vi "SCP_command_filtering.vi"(11 "Input":string) -> (3 "concatenated string":string)   [LabVIEW 2018, in "SCP.lvlib"]
uses:
  SCP.lvlib
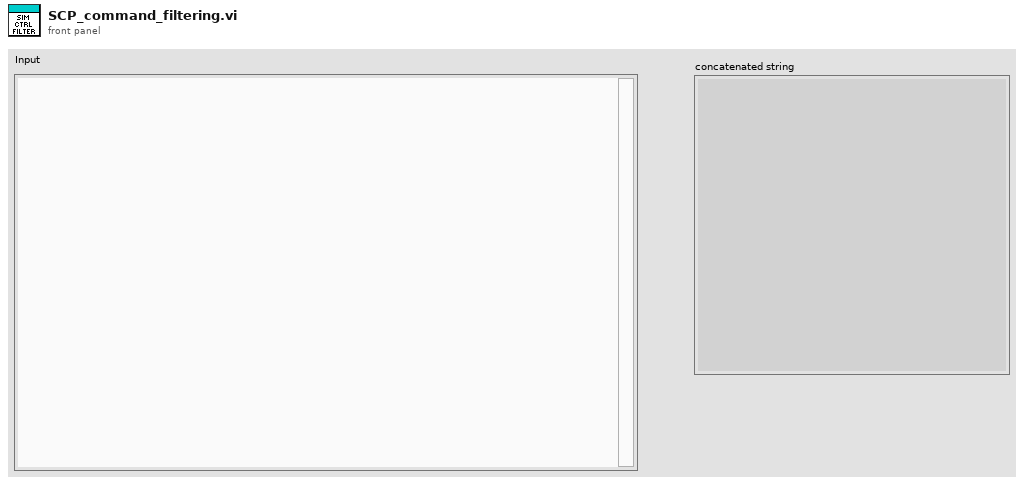
[diagram p1: front panel]
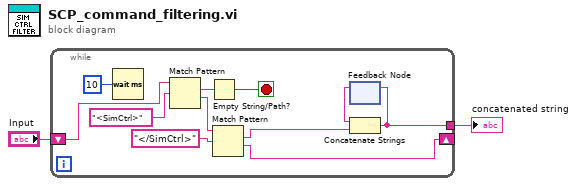
[diagram p0: block diagram]
diagram:
  n1 = while {
    shift-right: [w9] -> _
    shift-left: "Input" -> [w12]
    tunnel: [w6] -> w1
    stop <- w13 stop-if-true
    n2 = Wait (ms)(milliseconds to wait=u32 10) -> ()  [unwired: 1 out]
    n3 = Match Pattern(string=w12, regular expression="<SimCtrl>") -> (match substring=w11:string, after substring=w10:string)  [unwired: 1 in, 2 out]
    n4 = Empty String/Path?(string/path=w11) -> (empty?=w13:bool)
    n5 = Match Pattern(string=w10, regular expression="</SimCtrl>") -> (match substring=w3:string, after substring=w9:string)  [unwired: 1 in, 2 out]
    n6 = feedback #1() -> (w8:string)  [unwired: 1 in]
    n7 = Concatenate Strings(w8, w3) -> (w6:string)
    n8 = feedback-in #1(w6) -> ()
  }
  "concatenated string" <- w1
